vi "DMM.vi"() -> ()   [LabVIEW 2024]
uses:
  <vilib>/Analysis/baseanly.llb/Mean (DBL).vi
  EFmeter.lvlib
  <vilib>/Analysis/NI_AALBase.lvlib
panel:
  out "Waveform Graph":dbl[][](graph)
  out "Numeric 2":dbl
  out "Meter 2":dbl(knob) scale=0.0..5.0
  out "Numeric":dbl
  out "Meter":dbl(knob) scale=0.0..30.0
  in  "Clear":bool
  in  "Ulozit data":bool caption="Uložit data"
  in  "file path (use dialog)":path
  out "error out 2":errorcluster
  in  "EFmeter":refnum<visa-resource-name>
  in  "stop":bool
  in  "Start":bool
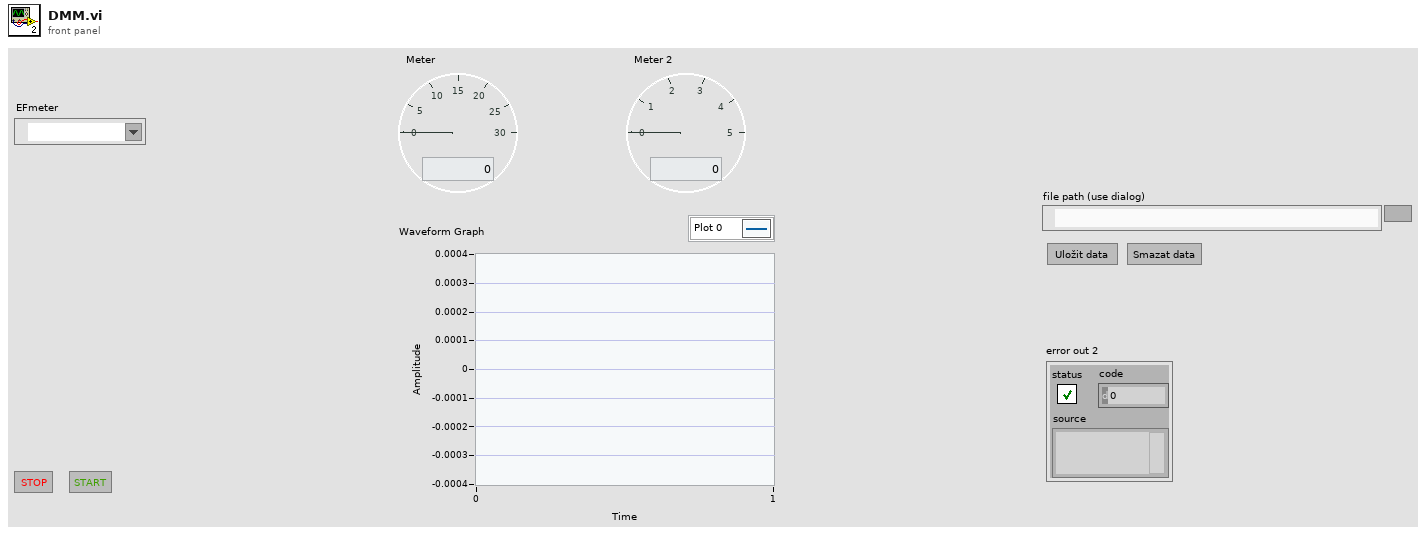
[diagram p1: front panel]
types:
  T1 = enum16{"open", "replace", "create", "open or create", "replace or create", "replace or create with confirmation"}
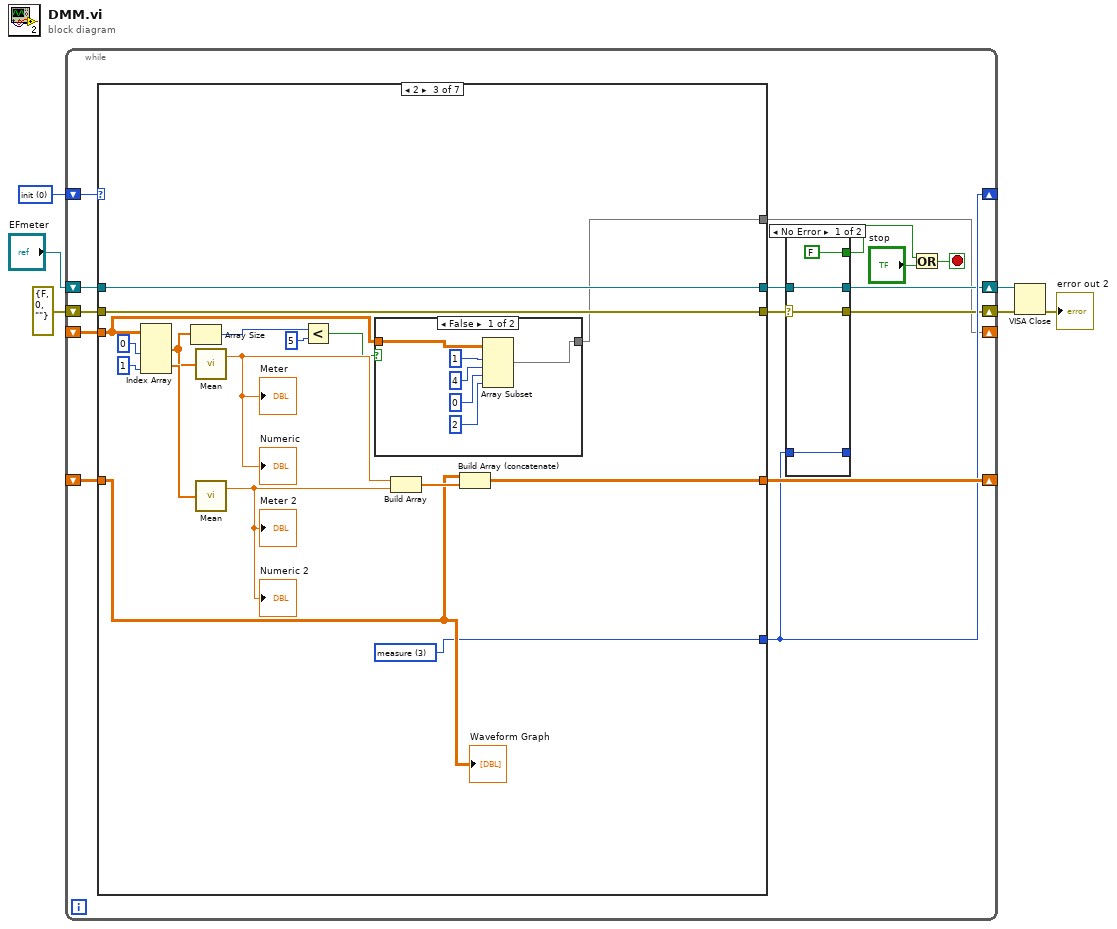
[diagram p0: block diagram]
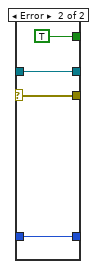
[diagram p2: hidden frame]
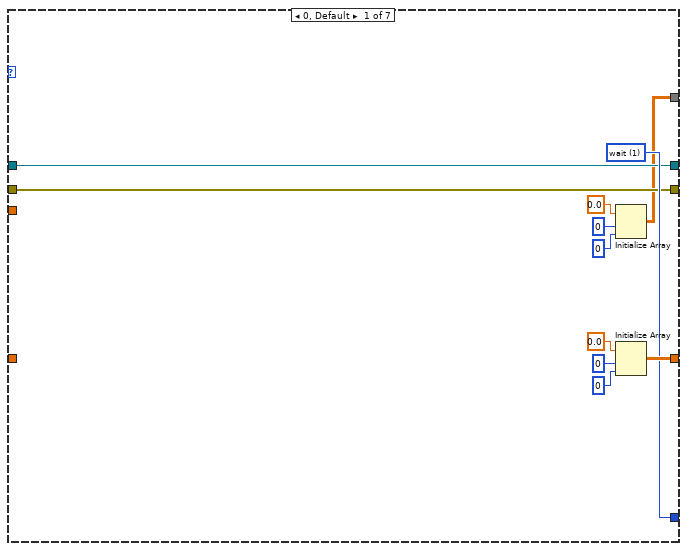
[diagram p3: hidden frame]
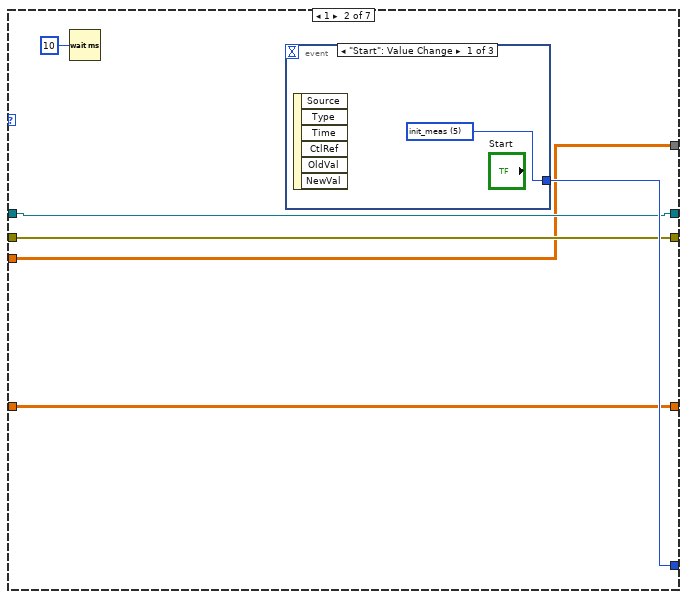
[diagram p4: hidden frame]
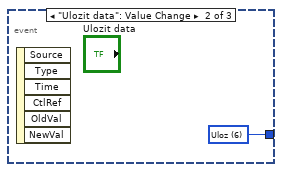
[diagram p5: hidden frame]
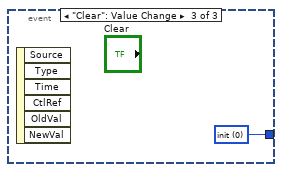
[diagram p6: hidden frame]
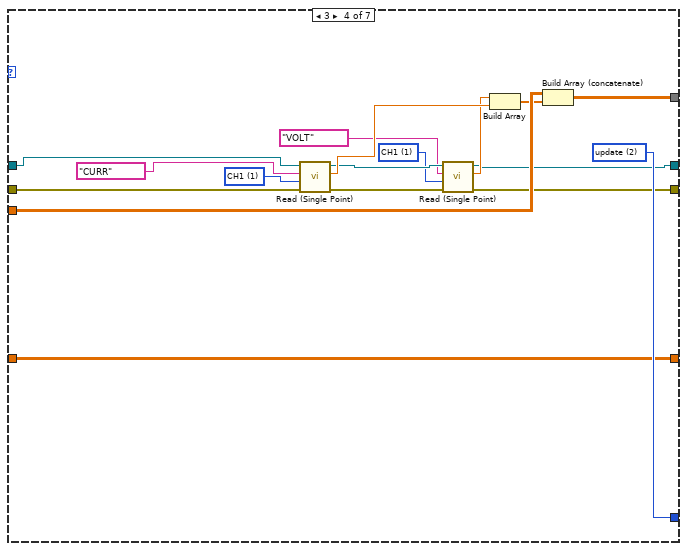
[diagram p8: hidden frame]
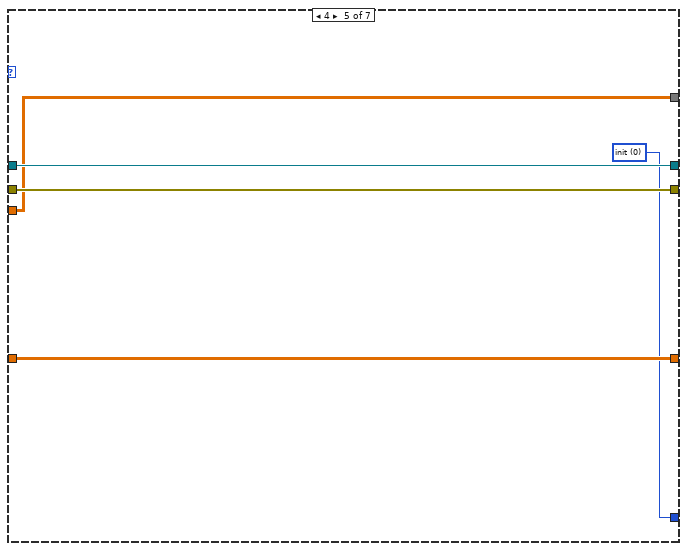
[diagram p9: hidden frame]
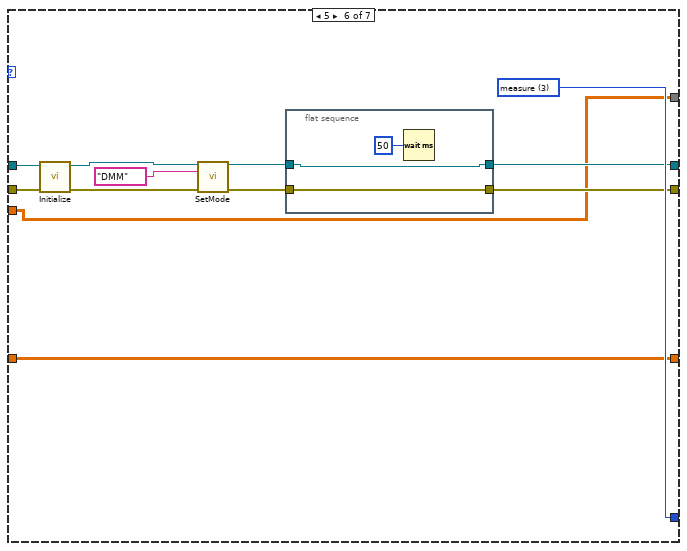
[diagram p10: hidden frame]
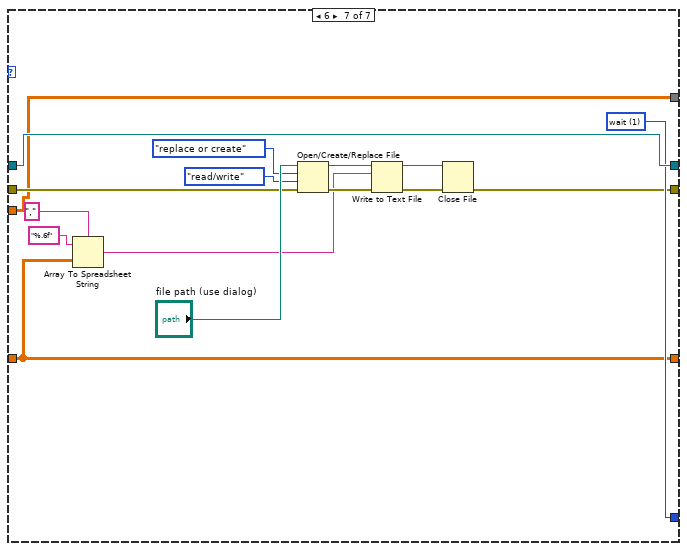
[diagram p11: hidden frame]
diagram:
  w6 = u16 0 items=["init", "wait", "update", "measure", "change_load", "init_meas", "Uloz", "clear"]
  n1 = while {
    shift-right: [w21] -> _
    shift-left: _ -> [w9]
    shift-right: [w17] -> _
    shift-left: w6 -> [w20]
    shift-right: [w14] -> w2
    shift-left: "EFmeter" -> [w19]
    shift-right: [w13] -> w1
    shift-left: errorcluster {"status"=FALSE, "code"=0, "source"=""} ("error in (no error)") -> [w18]
    shift-right: [w8] -> _
    shift-left: _ -> [w7]
    stop <- w11 stop-if-true
    n2 = case shown="2" w20 {
      tunnel: [w38 w42 w58 w74 w95 w97 w112] -> w21
      tunnel: [w37 w46 w50 w90 w92 w102 w120] -> w17
      tunnel: [w35 w44 w65 w76 w93 w99 w116] -> w16
      tunnel: [w34 w45 w66 w75 w94 w101 w126] -> w15
      tunnel: w19 -> [w34 w45 w66 w78 w94 w104 w126]
      tunnel: w18 -> [w35 w44 w65 w81 w93 w103 w122]
      tunnel: w9 -> [_ w42 w51 w74 w95 w97 w112]
      tunnel: [w30 w41 w56 w89 w91 w96 w111] -> w8
      tunnel: w7 -> [_ w41 w53 w88 w91 w96 w111]
      frame 0, Default {
        w37 = u16 1 items=["init", "wait", "update", "measure"]
        n3 = Initialize Array(0.0 ("element"), 0 ("dimension size"), 0 ("dimension size")) -> (w30:dbl[][])
        n4 = Initialize Array(0.0 ("element"), 0 ("dimension size"), 0 ("dimension size")) -> (w38:dbl[][])
      }
      frame 1 {
        n5 = Wait (ms)(milliseconds to wait=u32 10) -> ()  [unwired: 1 out]
        n6 = event shown="[0] \"Start\": Value Change" {
          selector: _ -> [_ _ _]
          dyn-events: _ -> [_ _ _]
          timeout: _ -> [_ _ _]
          tunnel: [w47 w48 w49] -> w46
          event "Start": Value Change {
            w47 = u16 5 items=["init", "wait", "update", "measure", "change_load", "init_meas"]
            n7 = event-data() -> ()  [unwired: 1 in, 6 out]
          }
          event "Ulozit data": Value Change {
            w48 = u16 6 items=["init", "wait", "update", "measure", "change_load", "init_meas", "Uloz"]
            n8 = event-data() -> ()  [unwired: 1 in, 6 out]
          }
          event "Clear": Value Change {
            w49 = u16 0 items=["init", "wait", "update", "measure", "change_load", "init_meas", "Uloz", "clear"]
            n9 = event-data() -> ()  [unwired: 1 in, 6 out]
          }
        }
      }
      frame 2 {
        w50 = u16 3 items=["init", "wait", "update", "measure"]
        n10 = Index Array(array=w53, index (col) #1=0 ("index (col)"), index (col) #2=1 ("index (col)")) -> (element #1=w57:dbl[], element #2=w62:dbl[])  [unwired: 2 in]
        n11 = Array Size(array=w57) -> (size(s)=w55:i32)
        n12 = call-poly <vilib>:"Mean.vi"("X"=w57) -> ("mean"=w61:dbl)  [unwired: 1 out]
        "Numeric" <- w61
        "Meter" <- w61
        n13 = call-poly <vilib>:"Mean.vi"("X"=w62) -> ("mean"=w60:dbl)  [unwired: 1 out]
        "Meter 2" <- w60
        "Numeric 2" <- w60
        n14 = Less?(x=w55, y=5) -> (x < y?=w52:bool)
        n15 = case shown="False" w52 {
          tunnel: w53 -> [w68 w73]
          tunnel: [w67 w73] -> w56
          frame False {
            n16 = Array Subset(array=w68, index (row)=1 ("index"), length (row)=4 ("length"), index (col)=0 ("index"), length (col)=2 ("length")) -> (w67:dbl[][])
          }
          frame True {
          }
        }
        n17 = Build Array(w61, w60) -> (w59:dbl[])
        n18 = Build Array (concatenate)(w51, w59) -> (w58:dbl[][])
        "Waveform Graph" <- w51
      }
      frame 3 {
        w80 = u16 1 items=["CH2"=2, "CH1"=1] ("Ring")
        w83 = u16 1 items=["CH2"=2, "CH1"=1] ("Ring")
        w90 = u16 2 items=["init", "wait", "update", "measure"]
        n19 = call "Read (Single Point).vi"("error in (no error)"=w81, "Ring"=w83, "Combo Box"="CURR", "VISA resource name"=w78) -> ("error out"=w84:errorcluster, "Measurement"=w87:dbl, "VISA resource name out"=w85:refnum<visa-resource-name>)  [unwired: 5 in]
        n20 = call "Read (Single Point).vi"("error in (no error)"=w84, "Ring"=w80, "Combo Box"="VOLT", "VISA resource name"=w85) -> ("error out"=w76:errorcluster, "Measurement"=w86:dbl, "VISA resource name out"=w75:refnum<visa-resource-name>)  [unwired: 5 in]
        n21 = Build Array(w86, w87) -> (w77:dbl[])
        n22 = Build Array (concatenate)(w88, w77) -> (w89:dbl[][])
      }
      frame 4 {
        w92 = u16 0 items=["init", "wait", "update", "measure", "change_load", "init_meas", "Uloz", "clear"]
      }
      frame 5 {
        w102 = u16 3 items=["init", "wait", "update", "measure", "change_load", "init_meas"]
        n23 = call "Initialize.vi"("error in (no error)"=w103, "VISA resource name"=w104) -> ("error out"=w107:errorcluster, "VISA resource name out"=w106:refnum<visa-resource-name>)  [unwired: 8 in]
        n24 = call "SetMode.vi"("VISA resource name"=w106, "Combo Box"="DMM", "error in (no error)"=w107) -> ("VISA resource name out"=w100:refnum<visa-resource-name>, "error out"=w98:errorcluster)  [unwired: 11 in]
        n25 = flat-sequence {
          tunnel: [w109] -> w101
          tunnel: w100 -> [w109]
          tunnel: w98 -> [w108]
          tunnel: [w108] -> w99
          frame #0 {
            n26 = Wait (ms)(milliseconds to wait=u32 50) -> ()  [unwired: 1 out]
          }
        }
      }
      frame 6 {
        w120 = u16 1 items=["init", "wait", "update", "measure", "change_load", "init_meas"]
        n27 = Array To Spreadsheet String(delimiter (Tab)=",", array=w112, 3:"%.6f" ("format string")) -> (spreadsheet string=w113:string)
        n28 = Open/Create/Replace File(file path (use dialog)="file path (use dialog)", error in=w122, operation (0:open)=T1."replace or create", access (0:read/write)=enum16{"read/write", "read-only", "write-only"}."read/write") -> (refnum out=w115:refnum<file>, error out=w118:errorcluster)  [unwired: 2 in, 1 out]
        n29 = Write to Text File(file (use dialog)=w115, text=w113, error in=w118) -> (refnum out=w114:refnum<file>, error out=w117:errorcluster)  [unwired: 1 in, 1 out]
        n30 = Close File(refnum=w114, error in=w117) -> (error out=w116:errorcluster)  [unwired: 1 out]
      }
    }
    n31 = case shown="No Error" w16 {
      selector: w16 -> [w23 w27]
      tunnel: w17 -> [w25 w28]
      tunnel: [w25 w28] -> _
      tunnel: w15 -> [w24 w29]
      tunnel: [w24 w29] -> w14
      tunnel: [w23 w27] -> w13
      tunnel: [FALSE TRUE] -> w10
      frame No Error {
      }
      frame Error {
      }
    }
    n32 = Or(x=w10, y="stop") -> (x .or. y?=w11:bool)
  }
  n33 = VISA Close(VISA resource name=w2, error in (no error)=w1) -> (error out=→"error out 2":errorcluster)
